vi "SeCrTs-Add_User .vi"(8 "error in (no error)":errorcluster) -> (0 "error out":errorcluster)   [LabVIEW 2022 SP3]
uses:
  <vilib>/Utility/error.llb/DialogType.ctl
  <vilib>/Utility/file.llb/Read Delimited Spreadsheet (string).vi
  <vilib>/Utility/file.llb/Write Delimited Spreadsheet (string).vi
panel:
  in  "BACK TO MAIN":bool
  in  "Access Level":u16(ring) items=["User", "Super User", "Admin"]
  in  "User Control":string[][](table)
  in  "Save":bool
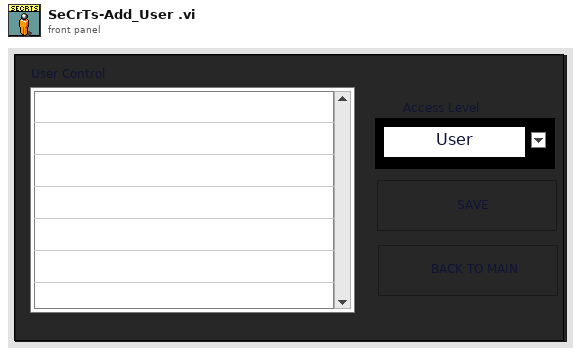
[diagram p1: front panel]
types:
  T1 = typedef "SeCrTs-file folder ctl.ctl" = cluster{"Datalog path":path, "Configuration path":path, "Signal list path":path, "Sub vi's":path, "Authentication":path, "Sequence":path, "Event Log":path, "CS Error log":path, "RT Error Log":path}
  T2 = typedef "LVRowAndColumnTypeDef.ctl" = cluster{"Row":i32, "Column":i32}
  T3 = typedef "DialogType.ctl" = u16
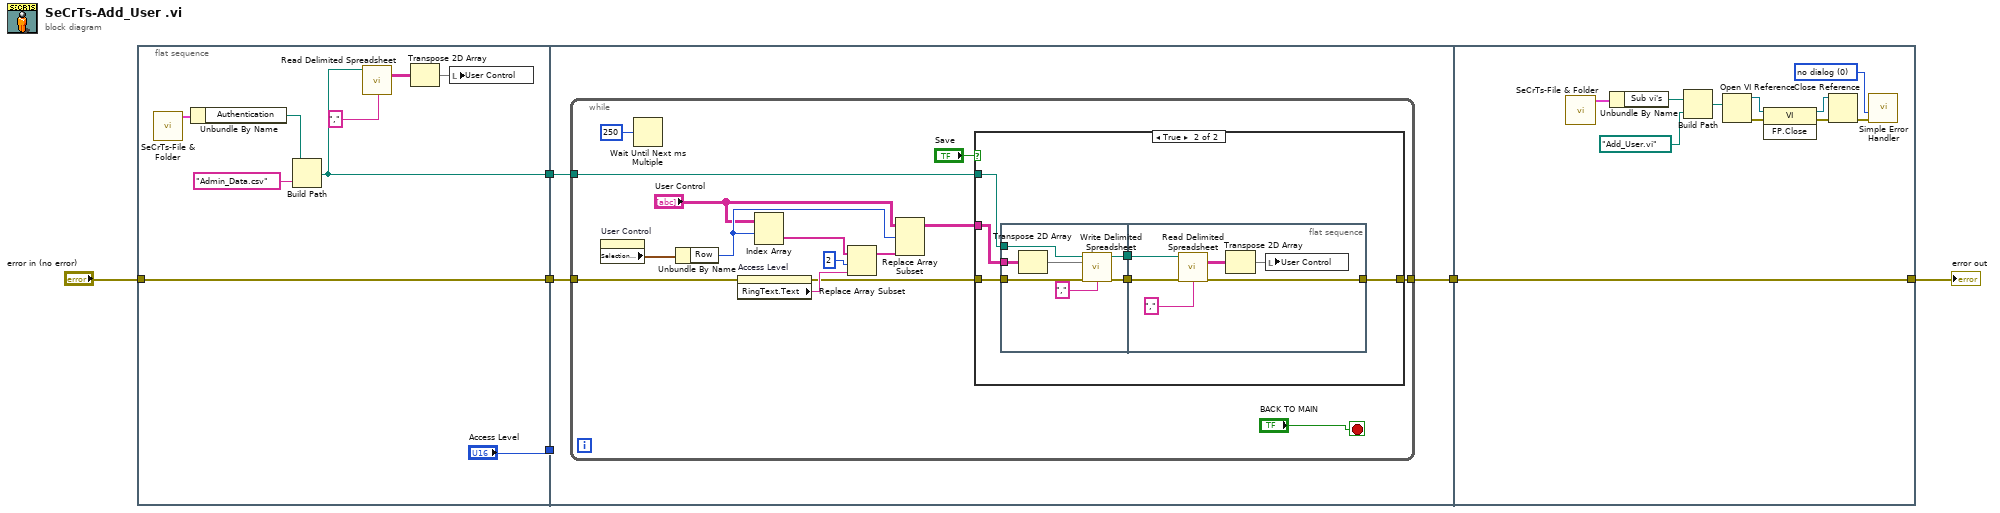
[diagram p0: block diagram]
diagram:
  n1 = flat-sequence {
    tunnel: ["Access Level"] -> w6
    tunnel: [w12] -> w5
    tunnel: "error in (no error)" -> [w9]
    tunnel: [w9] -> w4
    tunnel: w6 -> [_]
    tunnel: w5 -> [w18]
    tunnel: w4 -> [w17]
    tunnel: [w16] -> w1
    tunnel: [w64] -> w2
    tunnel: w1 -> [w64]
    frame #0 {
      n2 = call "SeCrTs-File & Folder.vi"() -> ("File Output"=w8:T1)  [unwired: 10 in, 1 out]
      n3 = Unbundle By Name(w8) -> ("Authentication"=w7:path)
      n4 = Build Path(base path=w7, name or relative path="Admin_Data.csv" ("name")) -> (appended path=w12:path)
      n5 = call-poly <vilib>:"Read Delimited Spreadsheet.vi"("file path (dialog if empty)"=w12, "delimiter (\\t)"="," ("delimiter (\\t)")) -> ("all rows"=w15:string[][])  [unwired: 8 in, 5 out]
      n6 = Transpose 2D Array(2D array=w15) -> (transposed array=w10:string[][])
      n7 = local write "User Control"(w10) -> ()
    }
    frame #1 {
      n8 = while {
        tunnel: w18 -> [w19]
        tunnel: w17 -> [w23]
        tunnel: [w21] -> w16
        stop <- "BACK TO MAIN" stop-if-true
        n9 = property on="User Control" class="Tbl (strict)"() -> ("Selection Start"=w33:T2)  [unwired: 2 in, 2 out]
        n10 = Wait Until Next ms Multiple(millisecond multiple=u32 250) -> ()  [unwired: 1 out]
        n11 = Unbundle By Name(w33) -> ("Row"=w31:i32)
        n12 = property on="Access Level" class="Ring (strict)"(error in=w23) -> (error out=w22:errorcluster, "RingText.Text"=w27:string)  [unwired: 1 in, 1 out]
        n13 = Index Array(array="User Control", index (row)=w31) -> (element=w30:string[])  [unwired: 1 in]
        n14 = Replace Array Subset(array=w30, new element=w27, index=2) -> (w28:string[])
        n15 = Replace Array Subset(array="User Control", new element=w28, index (row)=w31) -> (w32:string[][])  [unwired: 1 in]
        n16 = case shown="True" "Save" {
          tunnel: w32 -> [_ w40]
          tunnel: w19 -> [_ w39]
          tunnel: w22 -> [w34 w37]
          tunnel: [w34 w35] -> w21
          frame False {
          }
          frame True {
            n17 = flat-sequence {
              tunnel: w40 -> [w47]
              tunnel: w39 -> [w46]
              tunnel: [w44] -> w38
              tunnel: w37 -> [w42]
              tunnel: [w41] -> w36
              tunnel: w38 -> [w51]
              tunnel: w36 -> [w49]
              tunnel: [w48] -> w35
              frame #0 {
                n18 = Transpose 2D Array(2D array=w47) -> (transposed array=w45:string[][])
                n19 = call-poly <vilib>:"Write Delimited Spreadsheet.vi"("file path (dialog if empty)"=w46, "2D data"=w45, "error in (no error)"=w42, "delimiter (\\t)"="," ("delimiter (\\t)")) -> ("new file path (Not A Path if cancelled)"=w44:path, "error out"=w41:errorcluster)  [unwired: 10 in]
              }
              frame #1 {
                n20 = call-poly <vilib>:"Read Delimited Spreadsheet.vi"("file path (dialog if empty)"=w51, "error in (no error)"=w49, "delimiter (\\t)"="," ("delimiter (\\t)")) -> ("all rows"=w52:string[][], "error out"=w48:errorcluster)  [unwired: 7 in, 4 out]
                n21 = Transpose 2D Array(2D array=w52) -> (transposed array=w53:string[][])
                n22 = local write "User Control"(w53) -> ()
              }
            }
          }
        }
      }
    }
    frame #2 {
      w54 = T3 0 items=["no dialog", "OK message", "continue or stop message", "OK message + warnings", "continue/stop + warnings"] ("type of dialog (OK msg:1)")
      n23 = call "SeCrTs-File & Folder.vi"() -> ("File Output"=w61:T1)  [unwired: 10 in, 1 out]
      n24 = Unbundle By Name(w61) -> ("Sub vi's"=w60:path)
      n25 = Build Path(base path=w60, name or relative path=path "Add_User.vi") -> (appended path=w63:path)
      n26 = Open VI Reference(vi path=w63) -> (vi reference=w59:refnum<vi>, error out=w58:errorcluster)  [unwired: 5 in]
      n27 = invoke class="VI" method="FP.Close"(reference=w59, error in=w58) -> (reference out=w57:refnum<vi>, error out=w56:errorcluster)  [unwired: 1 in, 1 out]
      n28 = Close Reference(reference=w57, error in (no error)=w56) -> (error out=w55:errorcluster)
      n29 = call <vilib>:"Simple Error Handler.vi"("type of dialog (OK msg:1)"=w54, "error in (no error)"=w55) -> ()  [unwired: 3 in, 5 out]
    }
  }
  "error out" <- w2
